vi "Close.vi"(8 "error in":errorcluster, 11 "PCAN in":refnum<class "PCAN.lvclass">) -> (0 "error out":errorcluster, 3 "PCAN out":refnum<class "PCAN.lvclass">)   [LabVIEW 2023, in "PCAN.lvclass"]
uses:
  PCAN.lvclass
  PCAN.lvclass/PCAN.ctl
  Configurations/CFG JSON/CFG JSON.lvclass
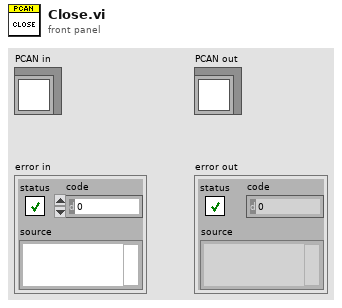
[diagram p1: front panel]
types:
  T1 = typedef "TPCANHandle.ctl" = enum16{"PCAN_NONEBUS  0x000", "PCAN_ISABUS1  0x21", "PCAN_ISABUS2  0x22", "PCAN_ISABUS3  0x23", "PCAN_ISABUS4  0x24", "PCAN_ISABUS5  0x25", "PCAN_ISABUS6  0x26", "PCAN_ISABUS7  0x27", "PCAN_ISABUS8  0x28", "PCAN_DNGBUS1  0x31", "PCAN_PCIBUS1  0x41", "PCAN_PCIBUS1  0x42", "PCAN_PCIBUS1  0x43", "PCAN_PCIBUS1  0x44", "PCAN_PCIBUS1  0x45", "PCAN_PCIBUS1  0x46", "PCAN_PCIBUS1  0x47", "PCAN_PCIBUS1  0x48", "PCAN_PCIBUS1  0x409", "PCAN_PCIBUS1  0x40A", "PCAN_PCIBUS1  0x40B", "PCAN_PCIBUS1  0x40C", "PCAN_PCIBUS1  0x40D", "PCAN_PCIBUS1  0x40E", "PCAN_PCIBUS1  0x40F", "PCAN_PCIBUS1  0x410", "PCAN_USBBUS1  0x51", "PCAN_USBBUS2  0x52", "PCAN_USBBUS3  0x53", "PCAN_USBBUS4  0x54", "PCAN_USBBUS5  0x55", "PCAN_USBBUS6  0x56", "PCAN_USBBUS7  0x57", "PCAN_USBBUS8  0x58", "PCAN_USBBUS9  0x509", "PCAN_USBBUS10  0x50A", "PCAN_USBBUS11  0x50B", "PCAN_USBBUS12  0x50C", "PCAN_USBBUS13  0x50D", "PCAN_USBBUS14  0x50E", "PCAN_USBBUS15  0x50F", "PCAN_USBBUS16  0x510", "PCAN_PCCBUS1  0x61", "PCAN_PCCBUS2  0x62", "PCAN_LANBUS1  0x801", "PCAN_LANBUS2  0x802", "PCAN_LANBUS3  0x803", "PCAN_LANBUS4  0x804", "PCAN_LANBUS5  0x805", "PCAN_LANBUS6  0x806", "PCAN_LANBUS7  0x807", "PCAN_LANBUS8  0x808", "PCAN_LANBUS9  0x809", "PCAN_LANBUS10  0x80A", "PCAN_LANBUS11  0x80B", "PCAN_LANBUS12  0x80C", "PCAN_LANBUS13  0x80D", "PCAN_LANBUS14  0x80E", "PCAN_LANBUS15  0x80F", "PCAN_LANBUS16  0x810"}
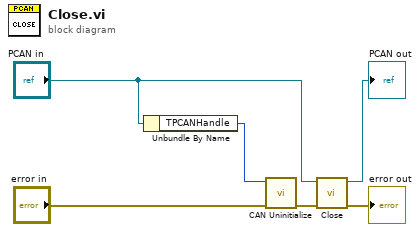
[diagram p0: block diagram]
diagram:
  n1 = Unbundle By Name("PCAN in") -> ("TPCANHandle"=w4:T1)
  n2 = call <instrlib>:"CAN Uninitialize.vi"("error in (no error)"="error in", "TPCANHandle"=w4) -> ("error out"=w5:errorcluster)  [unwired: 7 in, 2 out]
  n3 = call-parent "Close.vi"("error in"=w5, "CFG Base in"="PCAN in") -> ("error out"=→"error out":errorcluster, "CFG Base out"=→"PCAN out":refnum<class "PCAN.lvclass">)  [unwired: 8 in]
